vi "main2.vi"() -> ()   [LabVIEW 2020]
panel:
  in  "Numeric":dbl
  in  "String 2":string="123"
  out "String":string
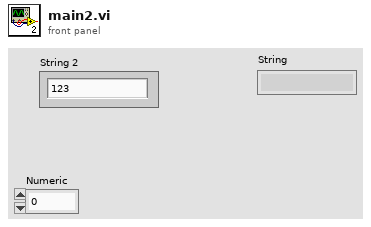
[diagram p1: front panel]
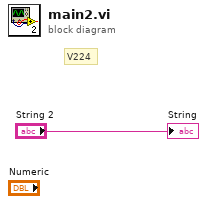
[diagram p0: block diagram]
diagram:
  # "V224"
  "String" <- "String 2"
